vi "Apply.vi"(8 "error in":errorcluster, 11 "Red-y Read Write CFG in":refnum<class "Red-y Read Write CFG.lvclass">) -> (0 "error out":errorcluster, 3 "Red-y Read Write CFG out":refnum<class "Red-y Read Write CFG.lvclass">)   [LabVIEW 2023, in "Red-y Read Write CFG.lvclass"]
uses:
  Red-y Read Write CFG.lvclass
  Red-y Read Write CFG.lvclass/Red-y Read Write CFG.ctl
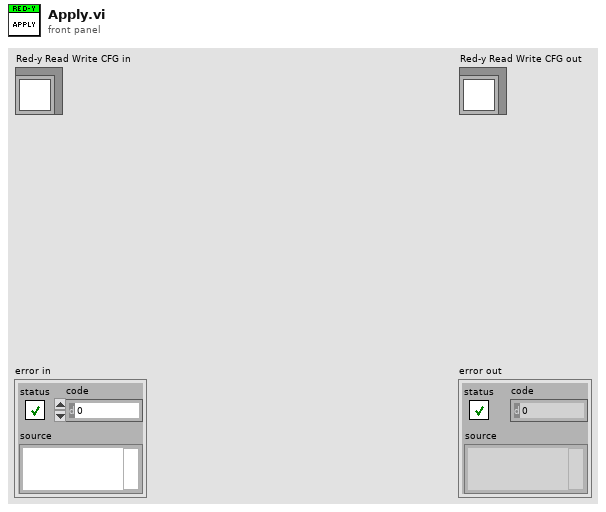
[diagram p1: front panel]
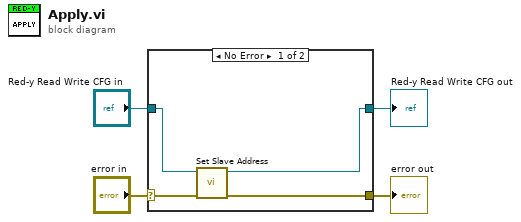
[diagram p0: block diagram]
diagram:
  n1 = case shown="No Error" "error in" {
    selector: "error in" -> [w8 w10]
    tunnel: [w7 w10] -> w3
    tunnel: [w5 w9] -> w1
    tunnel: "Red-y Read Write CFG in" -> [w6 w9]
    frame No Error {
      n2 = call-dynamic "Set Slave Address.vi"("error in"=w8, "Red-y Read Write CFG in"=w6) -> ("error out"=w7:errorcluster, "Red-y Read Write CFG out"=w5:refnum<class "Red-y Read Write CFG.lvclass">)  [unwired: 8 in]
    }
    frame Error {
    }
  }
  "error out" <- w3
  "Red-y Read Write CFG out" <- w1
